vi "Cleanup.vi"(8 "error in (no error)":errorcluster, 11 "Shared Options in":refnum<class "Shared Options.lvclass">) -> (0 "error out":errorcluster)   [LabVIEW 2020, in "AutoComplete.lvlib" / "Shared Options.lvclass"]
doc: "Cleans up the shared option instance. This should be done after all AutoComplete instances using the Shared Options have been closed otherwise they will no longer provide any options if still in use."
uses:
  Shared Options.lvclass
  Shared Options.lvclass/Shared Options.ctl
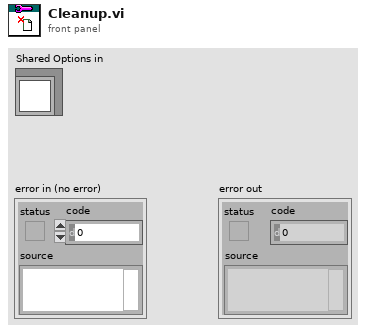
[diagram p1: front panel]
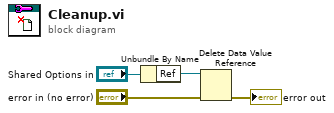
[diagram p0: block diagram]
diagram:
  n1 = Unbundle By Name("Shared Options in") -> ("Ref"=w3:refnum<data-value>)
  n2 = Delete Data Value Reference(data value reference=w3, error in="error in (no error)") -> (error out=→"error out":errorcluster)  [unwired: 1 out]
